vi "log analysis_gps.vi"() -> ()   [LabVIEW 2018] (continued)
41.292312622,-13.761383057,0.0,1.487377644,3.398363352,\"631T\",25,10,10,8,04,00,30,03*49b52b61\n\t", "INSPVAXA,USB3,0,44.5,FINESTEERING,2107,281284.250,02000000,471d,15824;INS_ALIGNMENT_COMPLETE,INS_RTKFIXED,37.37058446322,126.72127677415,9.0328,22.3000,0.3259,0.3273,-0.0037,-0.937814691,-0.658439283,39.092377906,0.4304,0.3133,0.6248,0.1182,0.0996,0.0951,0.2734,0.2534,5.0568,0f000001,0*6df0d0a0\n\t", "DUALANTENNAHEADINGA,USB3,0,45.0,FINESTEERING,2107,281285.200,02000000,d426,15824;SOL_COMPUTED,NARROW_INT,-1.000000000,40.100524902,-11.947021484,0.0,1.414593220,3.733982325,\"631T\",25,10,10,8,04,00,30,03*9b9ac519\n\t", "INSPVAXA,USB3,0,45.0,FINESTEERING,2107,281285.750,02000000,471d,15824;INS_ALIGNMENT_COMPLETE,INS_RTKFIXED,37.37058925318,126.72128198037,9.0239,22.3000,0.3334,0.2935,0.0143,-0.808488626,-0.666784324,37.099598741,0.4334,0.3188,0.6428,0.1170,0.0987,0.0941,0.2735,0.2534,5.0574,0f000001,0*332dca9d\n\t", "DUALANTENNAHEADINGA,USB3,0,47.0,FINESTEERING,2107,281286.700,02000000,d426,15824;SOL_COMPUTED,NARROW_INT,-1.000000000,38.718589783,-13.239685059,0.0,1.092944860,2.696835995,\"631T\",24,10,10,8,04,00,30,03*03484901\n\t", "DUALANTENNAHEADINGA,USB3,0,47.0,FINESTEERING,2107,281287.700,02000000,d426,15824;SOL_COMPUTED,NARROW_INT,-1.000000000,36.104297638,-13.498443604,0.0,0.922848761,2.195329189,\"631T\",26,10,10,8,04,00,30,03*04480a52\n\t", "INSPVAXA,USB3,0,47.5,FINESTEERING,2107,281288.250,02000000,471d,15824;INS_ALIGNMENT_COMPLETE,INS_RTKFIXED,37.37059781001,126.72128984433,9.0038,22.3000,0.3744,0.2594,-0.0022,-0.807848341,-0.697649833,32.607000206,0.4351,0.3197,0.6721,0.1156,0.0982,0.0924,0.2733,0.2531,5.0607,0f000001,0*7ad3d381\n\t", "DUALANTENNAHEADINGA,USB3,0,47.5,FINESTEERING,2107,281288.700,02000000,d426,15824;SOL_COMPUTED,NARROW_INT,-1.000000000,34.380798340,-12.289306641,0.0,0.881599903,2.027381897,\"631T\",24,10,10,8,04,00,30,03*fd23ace1\n\t", "INSPVAXA,USB3,0,43.0,FINESTEERING,2107,281289.250,02000000,471d,15824;INS_ALIGNMENT_COMPLETE,INS_RTKFIXED,37.37060144846,126.72129278207,8.9959,22.3000,0.3637,0.2540,-0.0055,-0.784801364,-1.198337190,31.676492197,0.4344,0.3185,0.6737,0.1148,0.0977,0.0905,0.2732,0.2529,5.0623,0f000001,0*0e64d244\n\t", "DUALANTENNAHEADINGA,USB3,0,47.0,FINESTEERING,2107,281290.200,02000000,d426,15824;SOL_COMPUTED,NARROW_INT,-1.000000000,34.493209839,-14.783813477,0.0,0.972535849,1.987741113,\"631T\",22,10,10,8,04,00,30,03*2d07aef6\n\t", "INSPVAXA,USB3,0,47.0,FINESTEERING,2107,281291.250,02000000,471d,15824;INS_ALIGNMENT_COMPLETE,INS_RTKFIXED,37.37060884718,126.72129871265,8.9767,22.3000,0.3938,0.2598,0.0143,-0.672164734,-1.279451684,31.580297519,0.4248,0.3046,0.6381,0.1143,0.0969,0.0864,0.2729,0.2527,5.0655,0f000001,0*eac27b45\n\t", "INSPVAXA,USB3,0,48.0,FINESTEERING,2107,281292.250,02000000,471d,15824;INS_ALIGNMENT_COMPLETE,INS_RTKFIXED,37.37061243778,126.72130169584,8.9693,22.3000,0.3929,0.2526,0.0002,-0.566566315,-1.022014825,31.866570439,0.4222,0.3014,0.6236,0.1151,0.0976,0.0859,0.2728,0.2526,5.0668,0f000001,0*f1faa83c\n\t", "INSPVAXA,USB3,0,46.5,FINESTEERING,2107,281293.250,02008000,471d,15824;INS_ALIGNMENT_COMPLETE,INS_RTKFIXED,37.37061609007,126.72130472150,8.9616,22.3000,0.3940,0.2710,0.0085,-0.635134028,-1.458627956,32.227180658,0.4201,0.2993,0.6101,0.1147,0.0971,0.0842,0.2727,0.2523,5.0683,0f000001,0*f561f230\n\t", "INSPVAXA,USB3,0,44.0,FINESTEERING,2107,281294.250,02008000,471d,15824;INS_ALIGNMENT_COMPLETE,INS_RTKFIXED,37.37061971209,126.72130780942,8.9541,22.3000,0.4211,0.2805,-0.0013,-0.831057528,-0.973116306,32.803325503,0.4188,0.2977,0.5988,0.1153,0.0975,0.0844,0.2725,0.2520,5.0696,0f000001,0*1928a823\n\t", "INSPVAXA,USB3,0,44.0,FINESTEERING,2107,281294.750,02008000,471d,15824;INS_ALIGNMENT_COMPLETE,INS_RTKFIXED,37.37062151019,126.72130936764,8.9520,22.3000,0.3975,0.2634,0.0090,-0.724790685,-1.060395947,33.026627760,0.4188,0.2977,0.5988,0.1153,0.0975,0.0844,0.2725,0.2520,5.0696,0f000001,0*daa7d020\n\t", "INSPVAXA,USB3,0,48.0,FINESTEERING,2107,281295.250,02008000,471d,15824;INS_ALIGNMENT_COMPLETE,INS_RTKFIXED,37.37062331676,126.72131094056,8.9508,22.3000,0.4136,0.2984,0.0031,-0.941558155,-1.233075222,33.345568477,0.4178,0.2964,0.5888,0.1164,0.0983,0.0857,0.2723,0.2516,5.0710,0f000001,0*4b91ac30\n\t", "INSPVAXA,USB3,0,48.0,FINESTEERING,2107,281295.750,02008000,471d,15824;INS_ALIGNMENT_COMPLETE,INS_RTKFIXED,37.37062507494,126.72131254716,8.9509,22.3000,0.4055,0.2849,-0.0018,-0.776132833,-1.125745955,33.718162525,0.4178,0.2964,0.5888,0.1164,0.0983,0.0857,0.2723,0.2516,5.0710,0f000001,0*fb568b3d\n\t", "INSPVAXA,USB3,0,46.0,FINESTEERING,2107,281296.750,02008000,471d,15824;INS_ALIGNMENT_COMPLETE,INS_RTKFIXED,37.37062859977,126.72131581022,8.9479,22.3000,0.4084,0.2870,-0.0048,-0.626858004,-1.220047276,34.496993035,0.4174,0.2953,0.5808,0.1166,0.0980,0.0866,0.2720,0.2512,5.0719,0f000001,0*b70d9a1a\n\t", "INSPVAXA,USB3,0,46.5,FINESTEERING,2107,281297.750,02000000,471d,15824;INS_ALIGNMENT_COMPLETE,INS_RTKFIXED,37.37063201269,126.72131910032,8.9415,22.3000,0.3858,0.2920,-0.0049,-0.857107455,-1.040274472,35.314316198,0.4170,0.2951,0.5749,0.1163,0.0975,0.0871,0.2718,0.2508,5.0734,0f000001,0*148bd1ed\n\t", "INSPVAXA,USB3,0,47.5,FINESTEERING,2107,281298.250,02000000,471d,15824;INS_ALIGNMENT_COMPLETE,INS_RTKFIXED,37.37063371305,126.72132080320,8.9374,22.3000,0.3749,0.3041,0.0076,-0.820490736,-1.287497218,35.568330559,0.4168,0.2950,0.5704,0.1159,0.0968,0.0877,0.2716,0.2505,5.0751,0f000001,0*0458b711\n\t", "INSPVAXA,USB3,0,48.0,FINESTEERING,2107,281299.250,02000000,471d,15824;INS_ALIGNMENT_COMPLETE,INS_RTKFIXED,37.37063695179,126.72132414290,8.9320,22.3000,0.3767,0.2972,0.0004,-0.739787726,-1.092581403,36.370475984,0.4162,0.2936,0.5661,0.1155,0.0962,0.0881,0.2714,0.2503,5.0767,0f000001,0*980b2911\n\t", "INSPVAXA,USB3,0,48.0,FINESTEERING,2107,281299.750,02000000,471d,15824;INS_ALIGNMENT_COMPLETE,INS_RTKFIXED,37.37063857725,126.72132585702,8.9270,22.3000,0.3719,0.3148,0.0043,-0.737895433,-1.223503382,36.673164573,0.4162,0.2936,0.5661,0.1155,0.0962,0.0881,0.2714,0.2503,5.0767,0f000001,0*b3e17f59\n\t", "INSPVAXA,USB3,0,49.0,FINESTEERING,2107,281300.750,02000000,471d,15824;INS_ALIGNMENT_COMPLETE,INS_RTKFIXED,37.37064174008,126.72132926537,8.9257,22.3000,0.3670,0.3118,0.0263,-0.579154984,-1.155742554,37.154805631,0.4158,0.2925,0.5630,0.1150,0.0956,0.0882,0.2713,0.2501,5.0783,0f000001,0*68bc3ddc\n\t", "INSPVAXA,USB3,0,45.0,FINESTEERING,2107,281301.250,02000000,471d,15824;INS_ALIGNMENT_COMPLETE,INS_RTKFIXED,37.37064333082,126.72133100341,8.9247,22.3000,0.3527,0.3031,-0.0127,-0.497881358,-1.036001571,37.376921117,0.4148,0.2915,0.5607,0.1142,0.0949,0.0876,0.2713,0.2501,5.0798,0f000001,0*cc5b3be5\n\t", "INSPVAXA,USB3,0,45.0,FINESTEERING,2107,281301.750,02000000,471d,15824;INS_ALIGNMENT_COMPLETE,INS_RTKFIXED,37.37064493780,126.72133275728,8.9253,22.3000,0.3854,0.3385,0.0182,-0.710763473,-1.064044201,37.431956874,0.4148,0.2915,0.5607,0.1142,0.0949,0.0876,0.2713,0.2501,5.0798,0f000001,0*85706bc5\n\t", "INSPVAXA,USB3,0,43.5,FINESTEERING,2107,281302.250,02000000,471d,15824;INS_ALIGNMENT_COMPLETE,INS_RTKFIXED,37.37064655535,126.72133453652,8.9249,22.3000,0.3513,0.3141,0.0174,-0.690110515,-1.069032412,37.638808056,0.4139,0.2898,0.5573,0.1136,0.0942,0.0868,0.2712,0.2501,5.0809,0f000001,0*cbae559e\n\t", "INSPVAXA,USB3,0,43.5,FINESTEERING,2107,281302.750,02000000,471d,15824;INS_ALIGNMENT_COMPLETE,INS_RTKFIXED,37.37064813520,126.72133627740,8.9245,22.3000,0.3692,0.3319,0.0061,-0.364312615,-0.951644319,37.470597230,0.4139,0.2898,0.5573,0.1136,0.0942,0.0868,0.2712,0.2501,5.0809,0f000001,0*08b0ee33\n\t", "INSPVAXA,USB3,0,47.5,FINESTEERING,2107,281303.750,02000000,471d,15824;INS_ALIGNMENT_COMPLETE,INS_RTKFIXED,37.37065132406,126.72133969488,8.9195,22.3000,0.3562,0.2992,-0.0320,-0.568216289,-0.963941072,36.278443582,0.4132,0.2892,0.5557,0.1134,0.0941,0.0862,0.2712,0.2500,5.0819,0f000001,0*4328ab23\n\t", "INSPVAXA,USB3,0,48.0,FINESTEERING,2107,281304.250,02000000,471d,15824;INS_ALIGNMENT_COMPLETE,INS_RTKFIXED,37.37065295180,126.72134135022,8.9157,22.3000,0.3763,0.3181,0.0214,-0.552058528,-1.148423815,35.386724637,0.4128,0.2880,0.5530,0.1133,0.0938,0.0856,0.2712,0.2500,5.0827,0f000001,0*325fffc2\n\t", "INSPVAXA,USB3,0,49.0,FINESTEERING,2107,281305.250,02000000,471d,15824;INS_ALIGNMENT_COMPLETE,INS_RTKFIXED,37.37065630183,126.72134454819,8.9059,22.3000,0.3906,0.3004,-0.0040,-0.611614094,-1.196662940,33.418986563,0.4115,0.2871,0.5504,0.1130,0.0936,0.0850,0.2711,0.2499,5.0838,0f000001,0*b360f959\n\t", "INSPVAXA,USB3,0,49.0,FINESTEERING,2107,281305.750,02000000,471d,15824;INS_ALIGNMENT_COMPLETE,INS_RTKFIXED,37.37065799694,126.72134610571,8.8988,22.3000,0.3773,0.2695,-0.0206,-0.928046219,-1.204880173,32.568917914,0.4115,0.2871,0.5504,0.1130,0.0936,0.0850,0.2711,0.2499,5.0838,0f000001,0*cfbde854\n\t", "INSPVAXA,USB3,0,43.0,FINESTEERING,2107,281306.750,02000000,471d,15824;INS_ALIGNMENT_COMPLETE,INS_RTKFIXED,37.37066149033,126.72134911698,8.8812,22.3000,0.3665,0.2586,0.0068,-0.726996907,-1.292564027,31.229501347,0.4104,0.2857,0.5476,0.1128,0.0935,0.0845,0.2710,0.2498,5.0853,0f000001,0*271f73c6\n\t", "INSPVAXA,USB3,0,47.5,FINESTEERING,2107,281307.250,02000000,471d,15824;INS_ALIGNMENT_COMPLETE,INS_RTKFIXED,37.37066326651,126.72135056496,8.8706,22.3000,0.3793,0.2759,-0.0087,-0.800097875,-1.188494571,30.825604162,0.4094,0.2846,0.5448,0.1127,0.0934,0.0841,0.2709,0.2497,5.0869,0f000001,0*7a768f4f\n\t", "INSPVAXA,USB3,0,47.5,FINESTEERING,2107,281307.750,02000000,471d,15824;INS_ALIGNMENT_COMPLETE,INS_RTKFIXED,37.37066506990,126.72135204695,8.8605,22.3000,0.3836,0.2569,-0.0181,-0.611818714,-1.092696034,30.573284565,0.4094,0.2846,0.5448,0.1127,0.0934,0.0841,0.2709,0.2497,5.0869,0f000001,0*79d635a4\n\t", "INSPVAXA,USB3,0,46.0,FINESTEERING,2107,281308.250,02000000,471d,15824;INS_ALIGNMENT_COMPLETE,INS_RTKFIXED,37.37066685186,126.72135349986,8.8501,22.3000,0.3922,0.2593,-0.0136,-0.551675825,-0.866778153,30.503806411,0.4391,0.2876,0.5552,0.1178,0.0942,0.0847,0.2709,0.2501,5.0885,0f000001,0*c2dc3b9a\n\t", "INSPVAXA,USB3,0,46.0,FINESTEERING,2107,281308.750,02000000,471d,15824;INS_ALIGNMENT_COMPLETE,INS_RTKFIXED,37.37066865801,126.72135498437,8.8428,22.3000,0.3889,0.2874,-0.0164,-0.422088252,-1.035305211,30.456393421,0.4391,0.2876,0.5552,0.1178,0.0942,0.0847,0.2709,0.2501,5.0885,0f000001,0*b848ab12\n\t", "INSPVAXA,USB3,0,48.0,FINESTEERING,2107,281309.750,02000000,471d,15824;INS_ALIGNMENT_COMPLETE,INS_RTKFIXED,37.37067230614,126.72135792146,8.8292,22.3000,0.4110,0.2664,-0.0105,-0.611662697,-1.081629993,30.781825564,0.4668,0.2909,0.5674,0.1216,0.0948,0.0853,0.2709,0.2504,5.0902,0f000001,0*6b834f48\n\t", "INSPVAXA,USB3,0,46.5,FINESTEERING,2107,281310.250,02000000,471d,15824;INS_ALIGNMENT_COMPLETE,INS_RTKFIXED,37.37067411015,126.72135939117,8.8212,22.3000,0.3810,0.2710,-0.0053,-0.603115000,-1.192069099,31.016227995,0.4406,0.2869,0.5568,0.1163,0.0939,0.0842,0.2707,0.2496,5.0919,0f000001,0*94346154\n\t", "INSPVAXA,USB3,0,46.5,FINESTEERING,2107,281310.750,02000000,471d,15824;INS_ALIGNMENT_COMPLETE,INS_RTKFIXED,37.37067588400,126.72136084983,8.8127,22.3000,0.4076,0.2839,-0.0115,-0.606845317,-1.152685391,31.227730506,0.4406,0.2869,0.5568,0.1163,0.0939,0.0842,0.2707,0.2496,5.0919,0f000001,0*103e46f3\n\t", "INSPVAXA,USB3,0,46.5,FINESTEERING,2107,281311.250,02000000,471d,15824;INS_ALIGNMENT_COMPLETE,INS_RTKFIXED,37.37067773364,126.72136238370,8.8047,22.3000,0.4077,0.2865,0.0068,-0.584908191,-1.091980758,31.544161154,0.4259,0.2849,0.5501,0.1143,0.0937,0.0835,0.2705,0.2492,5.0936,0f000001,0*c1eb006b\n\t", "INSPVAXA,USB3,0,46.5,FINESTEERING,2107,281311.750,02000000,471d,15824;INS_ALIGNMENT_COMPLETE,INS_RTKFIXED,37.37067959251,126.72136394573,8.7964,22.3000,0.4141,0.2904,-0.0295,-0.451303180,-1.068459528,31.726821051,0.4259,0.2849,0.5501,0.1143,0.0937,0.0835,0.2705,0.2492,5.0936,0f000001,0*f5652221\n\t", "INSPVAXA,USB3,0,48.5,FINESTEERING,2107,281312.250,02000000,471d,15824;INS_ALIGNMENT_COMPLETE,INS_RTKFIXED,37.37068138188,126.72136546046,8.7891,22.3000,0.3907,0.2897,-0.0164,-0.536773748,-1.064691543,31.954893776,0.4173,0.2841,0.5455,0.1136,0.0938,0.0834,0.2704,0.2490,5.0951,0f000001,0*3086f5e7\n\t", "INSPVAXA,USB3,0,48.5,FINESTEERING,2107,281312.750,02000000,471d,15824;INS_ALIGNMENT_COMPLETE,INS_RTKFIXED,37.37068318728,126.72136703307,8.7806,22.3000,0.4101,0.2924,-0.0105,-0.304454074,-0.851881109,32.302829580,0.4173,0.2841,0.5455,0.1136,0.0938,0.0834,0.2704,0.2490,5.0951,0f000001,0*5034c2f1\n\t", "INSPVAXA,USB3,0,45.5,FINESTEERING,2107,281314.250,02000000,471d,15824;INS_ALIGNMENT_COMPLETE,INS_RTKFIXED,37.37068860278,126.72137185474,8.7599,22.3000,0.3783,0.2883,-0.0099,-0.473451897,-1.199118445,33.419872159,0.4114,0.2852,0.5433,0.1126,0.0924,0.0813,0.2701,0.2485,5.0982,0f000001,0*254465a8\n\t", "INSPVAXA,USB3,0,45.5,FINESTEERING,2107,281314.750,02000000,471d,15824;INS_ALIGNMENT_COMPLETE,INS_RTKFIXED,37.37069038063,126.72137348955,8.7529,22.3000,0.4019,0.3010,-0.0013,-0.576554942,-1.350073245,33.962253064,0.4114,0.2852,0.5433,0.1126,0.0924,0.0813,0.2701,0.2485,5.0982,0f000001,0*70de1d9e\n\t", "INSPVAXA,USB3,0,50.0,FINESTEERING,2107,281316.250,02000000,471d,15824;INS_ALIGNMENT_COMPLETE,INS_RTKFIXED,37.37069553748,126.72137835296,8.7291,22.3000,0.3690,0.3016,-0.0165,-0.475362397,-1.709507066,35.267633649,0.4099,0.2844,0.5412,0.1123,0.0915,0.0796,0.2698,0.2480,5.0999,0f000001,0*7a9fb179\n\t", "INSPVAXA,USB3,0,50.5,FINESTEERING,2107,281317.250,02000000,471d,15824;INS_ALIGNMENT_COMPLETE,INS_RTKFIXED,37.37069888473,126.72138166049,8.7140,22.3000,0.4002,0.3322,-0.0336,-0.163313359,-1.347458535,36.032748786,0.4094,0.2836,0.5396,0.1129,0.0921,0.0802,0.2696,0.2478,5.0996,0f000001,0*7e476d51\n\t", "INSPVAXA,USB3,0,50.0,FINESTEERING,2107,281318.250,02000000,471d,15824;INS_ALIGNMENT_COMPLETE,INS_RTKFIXED,37.37070219067,126.72138499710,8.7014,22.3000,0.3959,0.3213,-0.0090,-0.394966992,-1.322496913,36.727773169,0.4088,0.2828,0.5369,0.1123,0.0917,0.0794,0.2695,0.2477,5.0989,0f000001,0*0ac65207\n\t", "INSPVAXA,USB3,0,48.5,FINESTEERING,2107,281319.750,02000000,471d,15824;INS_ALIGNMENT_COMPLETE,INS_RTKFIXED,37.37070705981,126.72139005862,8.6887,22.3000,0.3656,0.3184,-0.0246,-0.462020881,-1.503034844,37.411185291,0.4083,0.2820,0.5343,0.1120,0.0915,0.0787,0.2694,0.2475,5.0983,0f000001,0*abb76b38\n\t", "INSPVAXA,USB3,0,48.5,FINESTEERING,2107,281320.750,02000000,471d,15824;INS_ALIGNMENT_COMPLETE,INS_RTKFIXED,37.37071031528,126.72139346401,8.6801,22.3000,0.3719,0.3343,-0.0256,-0.836621928,-1.161971448,37.866051675,0.4083,0.2824,0.5333,0.1117,0.0916,0.0783,0.2693,0.2474,5.0979,0f000001,0*4c0e47a3\n\t", "INSPVAXA,USB3,0,47.0,FINESTEERING,2107,281322.250,02000000,471d,15824;INS_ALIGNMENT_COMPLETE,INS_RTKFIXED,37.37071517986,126.72139865405,8.6652,22.3000,0.3760,0.3375,-0.0171,-0.655763747,-1.033016654,37.379702834,0.4086,0.2835,0.5329,0.1123,0.0925,0.0785,0.2691,0.2470,5.0988,0f000001,0*f362831b\n\t", "INSPVAXA,USB3,0,48.5,FINESTEERING,2107,281323.750,02000000,471d,15824;INS_ALIGNMENT_COMPLETE,INS_RTKFIXED,37.37072004459,126.72140359087,8.6528,22.3000,0.3627,0.2855,-0.0006,-0.403703824,-0.919601594,35.267300347,0.4085,0.2834,0.5316,0.1119,0.0920,0.0781,0.2688,0.2467,5.1000,0f000001,0*ec9c6181\n\t", "INSPVAXA,USB3,0,48.0,FINESTEERING,2107,281350.300,02000000,471d,15824;INS_ALIGNMENT_COMPLETE,INS_RTKFIXED,37.37080986573,126.72148875740,8.5075,22.3000,0.3628,0.2976,-0.0057,-1.206867274,-0.983762536,33.908435264,0.4194,0.3028,0.5790,0.1129,0.0949,0.0832,0.2672,0.2431,5.1219,0f000001,0*073b2b30\n\t", "INSPVAXA,USB3,0,48.0,FINESTEERING,2107,281351.800,02000000,471d,15824;INS_ALIGNMENT_COMPLETE,INS_RTKFIXED,37.37081508694,126.72149360654,8.4972,22.3000,0.3531,0.2937,-0.0017,-1.250896951,-0.823004101,34.091002532,0.4207,0.3049,0.5833,0.1126,0.0947,0.0826,0.2672,0.2430,5.1224,0f000001,0*3c5ad9c3\n\t", "INSPVAXA,USB3,0,49.0,FINESTEERING,2107,281355.800,02000000,471d,15824;INS_ALIGNMENT_COMPLETE,INS_RTKFIXED,37.37082893700,126.72150664306,8.4666,22.3000,0.3730,0.3109,-0.0009,-1.161970784,-1.138060141,34.996264200,0.4190,0.3015,0.5793,0.1125,0.0944,0.0820,0.2670,0.2425,5.1250,0f000001,0*10c36a68\n\t", "INSPVAXA,USB3,0,48.0,FINESTEERING,2107,281356.300,02000000,471d,15824;INS_ALIGNMENT_COMPLETE,INS_RTKFIXED,37.37083063572,126.72150829045,8.4620,22.3000,0.3521,0.3106,-0.0162,-1.118678244,-0.900069608,35.100092302,0.4187,0.3015,0.5781,0.1134,0.0955,0.0834,0.2669,0.2424,5.1261,0f000001,0*ecce3653\n\t", "INSPVAXA,USB3,0,48.0,FINESTEERING,2107,281356.800,02000000,471d,15824;INS_ALIGNMENT_COMPLETE,INS_RTKFIXED,37.37083231067,126.72150995992,8.4554,22.3000,0.3495,0.3060,0.0042,-0.932722694,-0.812097133,35.195809963,0.4187,0.3015,0.5781,0.1134,0.0955,0.0834,0.2669,0.2424,5.1261,0f000001,0*f7e2c3ce\n\t", "INSPVAXA,USB3,0,47.5,FINESTEERING,2107,281358.300,02000000,471d,15824;INS_ALIGNMENT_COMPLETE,INS_RTKFIXED,37.37083738053,126.72151493365,8.4383,22.3000,0.3581,0.3251,0.0034,-0.998984174,-0.973141435,35.285574115,0.4158,0.2963,0.5677,0.1128,0.0943,0.0826,0.2668,0.2421,5.1287,0f000001,0*5ae881cd\n\t", "INSPVAXA,USB3,0,47.5,FINESTEERING,2107,281358.800,02000000,471d,15824;INS_ALIGNMENT_COMPLETE,INS_RTKFIXED,37.37083909479,126.72151662067,8.4311,22.3000,0.3558,0.3072,-0.0005,-0.868229023,-1.222380492,35.266513132,0.4158,0.2963,0.5677,0.1128,0.0943,0.0826,0.2668,0.2421,5.1287,0f000001,0*f5ce0274\n\t", "DUALANTENNAHEADINGA,USB3,0,49.0,FINESTEERING,2107,281360.300,02000000,d426,15824;SOL_COMPUTED,NARROW_FLOAT,-1.000000000,43.377029419,-28.936859131,0.0,317.200378418,180.000000000,\"631T\",19,9,9,8,04,00,20,03*d052c393\n\t", "DUALANTENNAHEADINGA,USB3,0,49.0,FINESTEERING,2107,281360.800,02000000,d426,15824;SOL_COMPUTED,NARROW_FLOAT,-1.000000000,41.997791290,-30.735473633,0.0,321.670349121,180.000000000,\"631T\",18,9,9,8,04,00,20,03*cef783d0\n\t", "DUALANTENNAHEADINGA,USB3,0,46.5,FINESTEERING,2107,281361.300,02000000,d426,15824;SOL_COMPUTED,NARROW_FLOAT,-1.000000000,39.328605652,-30.210357666,0.0,354.292755127,180.000000000,\"631T\",19,9,9,8,04,00,20,03*65c8eaaf\n\t", "INSPVAXA,USB3,0,46.5,FINESTEERING,2107,281361.800,02000000,471d,15824;INS_ALIGNMENT_COMPLETE,INS_RTKFIXED,37.37084928466,126.72152648987,8.4001,22.3000,0.3666,0.2894,0.0007,-0.918254878,-1.223429977,34.701580667,0.4179,0.3011,0.5737,0.1121,0.0941,0.0814,0.2668,0.2419,5.1323,0f000001,0*40ddb97a\n\t", "DUALANTENNAHEADINGA,USB3,0,48.0,FINESTEERING,2107,281362.300,02000000,d426,15824;SOL_COMPUTED,NARROW_FLOAT,-1.000000000,51.965854645,-24.394927979,0.0,236.640274048,180.000000000,\"631T\",19,9,9,8,04,00,20,03*62047533\n\t", "DUALANTENNAHEADINGA,USB3,0,48.0,FINESTEERING,2107,281362.800,02000000,d426,15824;SOL_COMPUTED,NARROW_FLOAT,-1.000000000,51.700309753,-22.485168457,0.0,233.081008911,180.000000000,\"631T\",19,9,9,8,04,00,20,03*ce0df6af\n\t", "DUALANTENNAHEADINGA,USB3,0,46.0,FINESTEERING,2107,281363.300,02000000,d426,15824;SOL_COMPUTED,NARROW_FLOAT,-1.000000000,37.930927277,-27.303833008,0.0,334.334472656,180.000000000,\"631T\",20,9,9,7,04,00,20,03*296cd207\n\t", "DUALANTENNAHEADINGA,USB3,0,46.0,FINESTEERING,2107,281363.800,02000000,d426,15824;SOL_COMPUTED,NARROW_FLOAT,-1.000000000,38.201625824,-27.727355957,0.0,332.017791748,180.000000000,\"631T\",23,9,9,8,04,00,20,03*f0493f23\n\t", "DUALANTENNAHEADINGA,USB3,0,44.0,FINESTEERING,2107,281364.300,02000000,d426,15824;SOL_COMPUTED,NARROW_FLOAT,-1.000000000,49.235725403,-25.915039063,0.0,256.086944580,180.000000000,\"631T\",24,9,9,8,04,00,20,03*6ae9d837\n\t", "INSPVAXA,USB3,0,44.0,FINESTEERING,2107,281364.800,02000000,471d,15824;INS_ALIGNMENT_COMPLETE,INS_RTKFIXED,37.37085965164,126.72153621397,8.3672,22.3000,0.3702,0.3004,-0.0120,-0.629392429,-1.475289805,34.330847261,0.4175,0.2991,0.5747,0.1118,0.0936,0.0803,0.2665,0.2416,5.1319,0f000001,0*907d57c4\n\t", "DUALANTENNAHEADINGA,USB3,0,48.0,FINESTEERING,2107,281365.300,02000000,d426,15824;SOL_COMPUTED,NARROW_FLOAT,-1.000000000,46.742221832,-24.611022949,0.0,308.216918945,180.000000000,\"631T\",18,9,9,8,04,00,20,03*16f83fc7\n\t", "DUALANTENNAHEADINGA,USB3,0,48.0,FINESTEERING,2107,281365.800,02000000,d426,15824;SOL_COMPUTED,NARROW_FLOAT,-1.000000000,45.876544952,-25.206176758,0.0,301.727966309,180.000000000,\"631T\",19,9,9,8,04,00,20,03*878e3cfa\n\t", "INSPVAXA,USB3,0,50.0,FINESTEERING,2107,281366.300,02000000,471d,15824;INS_ALIGNMENT_COMPLETE,INS_RTKFIXED,37.37086481879,126.72154103574,8.3492,22.3000,0.3841,0.2933,-0.0130,-0.540868347,-1.307063717,34.323850336,0.4168,0.2979,0.5715,0.1114,0.0932,0.0794,0.2664,0.2414,5.1301,0f000001,0*c00b2394\n\t", "INSPVAXA,USB3,0,50.0,FINESTEERING,2107,281366.800,02000000,471d,15824;INS_ALIGNMENT_COMPLETE,INS_RTKFIXED,37.37086653652,126.72154262606,8.3447,22.3000,0.3779,0.3041,-0.0177,-0.586317091,-1.274041965,34.268661727,0.4168,0.2979,0.5715,0.1114,0.0932,0.0794,0.2664,0.2414,5.1301,0f000001,0*197e2cdd\n\t", "DUALANTENNAHEADINGA,USB3,0,48.0,FINESTEERING,2107,281367.300,02000000,d426,15824;SOL_COMPUTED,NARROW_FLOAT,-1.000000000,57.061241150,-31.246337891,0.0,140.264724731,180.000000000,\"631T\",19,11,11,8,04,00,30,03*83af5acf\n\t", "DUALANTENNAHEADINGA,USB3,0,48.0,FINESTEERING,2107,281367.800,02000000,d426,15824;SOL_COMPUTED,NARROW_FLOAT,-1.000000000,57.968719482,-32.427215576,0.0,139.111709595,180.000000000,\"631T\",22,11,11,8,04,00,30,03*64b77029\n\t", "INSPVAXA,USB3,0,45.0,FINESTEERING,2107,281368.300,02000000,471d,15824;INS_ALIGNMENT_COMPLETE,INS_RTKFIXED,37.37087168794,126.72154735160,8.3372,22.3000,0.3761,0.3168,-0.0092,-0.837699273,-0.815511230,34.270342618,0.4149,0.2944,0.5637,0.1114,0.0930,0.0792,0.2662,0.2411,5.1296,0f000001,0*cf514333\n\t", "INSPVAXA,USB3,0,45.0,FINESTEERING,2107,281368.800,02000000,471d,15824;INS_ALIGNMENT_COMPLETE,INS_RTKFIXED,37.37087344572,126.72154897754,8.3331,22.3000,0.3716,0.2920,0.0040,-0.667583562,-0.920128671,34.279798590,0.4149,0.2944,0.5637,0.1114,0.0930,0.0792,0.2662,0.2411,5.1296,0f000001,0*f456fa2a\n\t", "DUALANTENNAHEADINGA,USB3,0,47.0,FINESTEERING,2107,281369.300,02000000,d426,15824;SOL_COMPUTED,NARROW_FLOAT,-1.000000000,48.869911194,-23.291656494,0.0,246.362884521,180.000000000,\"631T\",19,9,9,8,04,00,20,03*fdb2b4cf\n\t", "INSPVAXA,USB3,0,47.0,FINESTEERING,2107,281369.800,02000000,471d,15824;INS_ALIGNMENT_COMPLETE,INS_RTKFIXED,37.37087693639,126.72155218192,8.3258,22.3000,0.3824,0.3082,-0.0032,-0.585559020,-1.104223780,34.420056753,0.4144,0.2935,0.5605,0.1112,0.0927,0.0788,0.2662,0.2410,5.1304,0f000001,0*fed5d425\n\t", "DUALANTENNAHEADINGA,USB3,0,48.5,FINESTEERING,2107,281370.300,02000000,d426,15824;SOL_COMPUTED,NARROW_FLOAT,-1.000000000,56.995876312,-45.029174805,0.0,226.826354980,180.000000000,\"631T\",18,8,8,8,04,00,20,03*06abc766\n\t", "DUALANTENNAHEADINGA,USB3,0,48.5,FINESTEERING,2107,281370.800,02000000,d426,15824;SOL_COMPUTED,NARROW_FLOAT,-1.000000000,56.755435944,-45.314361572,0.0,225.346038818,180.000000000,\"631T\",19,8,8,8,04,00,20,03*c8312a5e\n\t", "DUALANTENNAHEADINGA,USB3,0,47.5,FINESTEERING,2107,281371.800,02000000,d426,15824;SOL_COMPUTED,NARROW_FLOAT,-1.000000000,65.830406189,-48.192810059,0.0,160.190460205,180.000000000,\"631T\",20,8,8,8,04,00,20,03*a1e2e423\n\t", "DUALANTENNAHEADINGA,USB3,0,51.0,FINESTEERING,2107,281372.300,02000000,d426,15824;SOL_COMPUTED,NARROW_FLOAT,-1.000000000,46.303096771,-16.665802002,0.0,249.117385864,180.000000000,\"631T\",21,9,9,8,04,00,20,03*9ebf37bc\n\t", "DUALANTENNAHEADINGA,USB3,0,51.0,FINESTEERING,2107,281372.800,02000000,d426,15824;SOL_COMPUTED,NARROW_FLOAT,-1.000000000,47.137203217,-16.407073975,0.0,245.953109741,180.000000000,\"631T\",21,9,9,8,04,00,20,03*e468614e\n\t", "DUALANTENNAHEADINGA,USB3,0,48.0,FINESTEERING,2107,281373.300,02000000,d426,15824;SOL_COMPUTED,NARROW_FLOAT,-1.000000000,40.694911957,-17.624786377,0.0,282.511657715,180.000000000,\"631T\",21,9,9,8,04,00,20,03*fc4a9f69\n\t", "DUALANTENNAHEADINGA,USB3,0,48.0,FINESTEERING,2107,281373.800,02000000,d426,15824;SOL_COMPUTED,NARROW_FLOAT,-1.000000000,39.396804810,-18.797271729,0.0,283.153411865,180.000000000,\"631T\",22,9,9,8,04,00,20,03*8a178ec6\n\t", "DUALANTENNAHEADINGA,USB3,0,45.0,FINESTEERING,2107,281374.800,02000000,d426,15824;SOL_COMPUTED,NARROW_FLOAT,-1.000000000,39.349189758,-20.650939941,0.0,277.168212891,180.000000000,\"631T\",22,9,9,8,04,00,20,03*f8ab3252\n\t", "DUALANTENNAHEADINGA,USB3,0,44.5,FINESTEERING,2107,281375.300,02000000,d426,15824;SOL_COMPUTED,NARROW_FLOAT,-1.000000000,34.529243469,-20.115325928,0.0,317.339965820,180.000000000,\"631T\",22,9,9,8,04,00,20,03*a594d36f\n\t", "DUALANTENNAHEADINGA,USB3,0,44.5,FINESTEERING,2107,281375.800,02000000,d426,15824;SOL_COMPUTED,NARROW_FLOAT,-1.000000000,34.753417969,-19.800323486,0.0,315.846893311,180.000000000,\"631T\",22,9,9,8,04,00,20,03*6b0303b2\n\t", "DUALANTENNAHEADINGA,USB3,0,46.0,FINESTEERING,2107,281376.300,02000000,d426,15824;SOL_COMPUTED,NARROW_FLOAT,-1.000000000,41.617706299,-20.286529541,0.0,249.996673584,180.000000000,\"631T\",22,9,9,8,04,00,20,03*8e0e78c9\n\t", "DUALANTENNAHEADINGA,USB3,0,45.0,FINESTEERING,2107,281377.300,02000000,d426,15824;SOL_COMPUTED,NARROW_FLOAT,-1.000000000,38.012714386,-20.573577881,0.0,307.964691162,180.000000000,\"631T\",20,9,9,8,04,00,20,03*3937b18a\n\t", "DUALANTENNAHEADINGA,USB3,0,45.0,FINESTEERING,2107,281377.800,02000000,d426,15824;SOL_COMPUTED,NARROW_FLOAT,-1.000000000,38.498992920,-20.027069092,0.0,303.899200439,180.000000000,\"631T\",20,9,9,8,04,00,20,03*e32a34d5\n\t", "DUALANTENNAHEADINGA,USB3,0,49.5,FINESTEERING,2107,281378.300,02000000,d426,15824;SOL_COMPUTED,NARROW_FLOAT,-1.000000000,27.239126205,-17.903564453,0.0,360.000000000,180.000000000,\"631T\",20,9,9,8,04,00,20,03*3fff5ac6\n\t", "DUALANTENNAHEADINGA,USB3,0,48.5,FINESTEERING,2107,281379.300,02000000,d426,15824;SOL_COMPUTED,NARROW_FLOAT,-1.000000000,30.153203964,-39.951202393,0.0,341.163116455,180.000000000,\"631T\",22,8,8,8,04,00,20,03*fe3aefcd\n\t", "DUALANTENNAHEADINGA,USB3,0,47.5,FINESTEERING,2107,281380.300,02000000,d426,15824;SOL_COMPUTED,NARROW_FLOAT,-1.000000000,31.592365265,-19.809661865,0.0,316.837921143,180.000000000,\"631T\",19,9,9,8,04,00,20,03*09fa2adc\n\t", "DUALANTENNAHEADINGA,USB3,0,46.0,FINESTEERING,2107,281381.300,02000000,d426,15824;SOL_COMPUTED,NARROW_FLOAT,-1.000000000,31.278856277,-21.390625000,0.0,327.912139893,180.000000000,\"631T\",19,9,9,8,04,00,20,03*4fc11f4c\n\t", "INSPVAXA,USB3,0,46.0,FINESTEERING,2107,281381.850,02000000,471d,15824;INS_ALIGNMENT_COMPLETE,INS_RTKFIXED,37.37091780548,126.72159081675,8.2350,22.3000,0.3759,0.2927,0.0016,-0.963689803,-1.123540768,33.630773348,0.4181,0.3018,0.5653,0.1129,0.0953,0.0850,0.2661,0.2404,5.1482,0f000001,0*05f2b425\n\t", "DUALANTENNAHEADINGA,USB3,0,49.5,FINESTEERING,2107,281382.800,02000000,d426,15824;SOL_COMPUTED,NARROW_FLOAT,-1.000000000,34.756454468,-17.411163330,0.0,292.158599854,180.000000000,\"631T\",19,9,9,8,04,00,20,03*833ed280\n\t", "DUALANTENNAHEADINGA,USB3,0,48.0,FINESTEERING,2107,281383.300,02000000,d426,15824;SOL_COMPUTED,NARROW_FLOAT,-1.000000000,29.882240295,-12.166564941,0.0,299.295318604,180.000000000,\"631T\",20,9,9,8,04,00,20,03*2118f19e\n\t", "INSPVAXA,USB3,0,48.0,FINESTEERING,2107,281383.850,02000000,471d,15824;INS_ALIGNMENT_COMPLETE,INS_RTKFIXED,37.37092469082,126.72159717751,8.2117,22.3000,0.3710,0.2982,-0.0132,-1.063340683,-1.217564676,33.617373330,0.4191,0.3013,0.5725,0.1134,0.0950,0.0851,0.2661,0.2404,5.1497,0f000001,0*b9a6888a\n\t", "INSPVAXA,USB3,0,49.0,FINESTEERING,2107,281385.350,02000000,471d,15824;INS_ALIGNMENT_COMPLETE,INS_RTKFIXED,37.37092984687,126.72160192884,8.2009,22.3000,0.3659,0.2906,-0.0108,-0.966416737,-0.773960288,33.451430049,0.4185,0.2991,0.5729,0.1134,0.0948,0.0848,0.2660,0.2403,5.1498,0f000001,0*c2089fa9\n\t", "INSPVAXA,USB3,0,49.0,FINESTEERING,2107,281385.850,02000000,471d,15824;INS_ALIGNMENT_COMPLETE,INS_RTKFIXED,37.37093156972,126.72160349245,8.1991,22.3000,0.3552,0.2819,0.0017,-0.982402524,-0.987093830,33.457221519,0.4185,0.2991,0.5729,0.1134,0.0948,0.0848,0.2660,0.2403,5.1498,0f000001,0*8db597c9\n\t", "INSPVAXA,USB3,0,46.0,FINESTEERING,2107,281386.850,02000000,471d,15824;INS_ALIGNMENT_COMPLETE,INS_RTKFIXED,37.37093500656,126.72160657159,8.1978,22.3000,0.3860,0.2986,-0.0065,-0.930872832,-0.693352418,33.361120344,0.4182,0.2979,0.5715,0.1134,0.0948,0.0846,0.2660,0.2403,5.1494,0f000001,0*a8ec127a\n\t", "INSPVAXA,USB3,0,48.5,FINESTEERING,2107,281387.850,02000000,471d,15824;INS_ALIGNMENT_COMPLETE,INS_RTKFIXED,37.37093847805,126.72160977606,8.1934,22.3000,0.3545,0.2733,-0.0290,-0.871913936,-1.019858036,33.407520693,0.4181,0.2974,0.5707,0.1132,0.0948,0.0844,0.2660,0.2403,5.1492,0f000001,0*8b26d1b5\n\t", "INSPVAXA,USB3,0,47.0,FINESTEERING,2107,281388.850,02000000,471d,15824;INS_ALIGNMENT_COMPLETE,INS_RTKFIXED,37.37094185798,126.72161284652,8.1862,22.3000,0.3458,0.2807,0.0000,-0.647146834,-0.755815505,33.229882391,0.4177,0.2968,0.5693,0.1134,0.0951,0.0842,0.2659,0.2403,5.1493,0f000001,0*e04b9d7e\n\t", "INSPVAXA,USB3,0,51.0,FINESTEERING,2107,281389.850,02000000,471d,15824;INS_ALIGNMENT_COMPLETE,INS_RTKFIXED,37.37094531152,126.72161597043,8.1814,22.3000,0.3770,0.3007,-0.0075,-0.964998734,-0.610692019,33.331132112,0.4178,0.2983,0.5697,0.1133,0.0955,0.0841,0.2659,0.2402,5.1491,0f000001,0*f3e7f4f6\n\t", "INSPVAXA,USB3,0,50.5,FINESTEERING,2107,281390.350,02000000,471d,15824;INS_ALIGNMENT_COMPLETE,INS_RTKFIXED,37.37094699615,126.72161749721,8.1810,22.3000,0.3585,0.2781,-0.0176,-0.963426361,-0.735868518,33.269975778,0.4179,0.2987,0.5691,0.1132,0.0952,0.0837,0.2658,0.2402,5.1481,0f000001,0*d9e47fdc\n\t", "INSPVAXA,USB3,0,50.5,FINESTEERING,2107,281390.850,02000000,471d,15824;INS_ALIGNMENT_COMPLETE,INS_RTKFIXED,37.37094874032,126.72161908849,8.1805,22.3000,0.3294,0.2293,-0.0009,-0.908401670,-0.595727338,33.364278854,0.4179,0.2987,0.5691,0.1132,0.0952,0.0837,0.2658,0.2402,5.1481,0f000001,0*5999a9d2\n\t", "INSPVAXA,USB3,0,48.0,FINESTEERING,2107,281391.350,02000000,471d,15824;INS_ALIGNMENT_COMPLETE,INS_RTKFIXED,37.37095049924,126.72162069173,8.1796,22.3000,0.4034,0.3085,-0.0112,-0.795383493,-0.971346032,33.378242699,0.4182,0.2986,0.5686,0.1132,0.0949,0.0836,0.2658,0.2402,5.1464,0f000001,0*1e48eff8\n\t", "INSPVAXA,USB3,0,48.0,FINESTEERING,2107,281391.850,02000000,471d,15824;INS_ALIGNMENT_COMPLETE,INS_RTKFIXED,37.37095218768,126.72162223158,8.1782,22.3000,0.3736,0.3039,0.0085,-0.869440972,-1.042554722,33.323263236,0.4182,0.2986,0.5686,0.1132,0.0949,0.0836,0.2658,0.2402,5.1464,0f000001,0*be662b3c\n\t", "INSPVAXA,USB3,0,46.5,FINESTEERING,2107,281392.850,02000000,471d,15824;INS_ALIGNMENT_COMPLETE,INS_RTKFIXED,37.37095563956,126.72162543709,8.1738,22.3000,0.3750,0.2874,-0.0042,-0.381103782,-1.196591916,33.536451772,0.4182,0.2976,0.5666,0.1131,0.0944,0.0833,0.2657,0.2401,5.1446,0f000001,0*fd2c5164\n\t", "INSPVAXA,USB3,0,47.0,FINESTEERING,2107,281393.350,02000000,471d,15824;INS_ALIGNMENT_COMPLETE,INS_RTKFIXED,37.37095732903,126.72162695963,8.1710,22.3000,0.3684,0.2951,-0.0131,-0.615904330,-1.127921907,33.544859726,0.4171,0.2952,0.5633,0.1132,0.0946,0.0833,0.2656,0.2401,5.1445,0f000001,0*dbe231da\n\t", "INSPVAXA,USB3,0,47.0,FINESTEERING,2107,281393.850,02000000,471d,15824;INS_ALIGNMENT_COMPLETE,INS_RTKFIXED,37.37095908537,126.72162857603,8.1657,22.3000,0.3533,0.2801,-0.0216,-0.431209048,-1.265989093,33.662345403,0.4171,0.2952,0.5633,0.1132,0.0946,0.0833,0.2656,0.2401,5.1445,0f000001,0*22a3a0dc\n\t", "INSPVAXA,USB3,0,49.5,FINESTEERING,2107,281394.350,02000000,471d,15824;INS_ALIGNMENT_COMPLETE,INS_RTKFIXED,37.37096076368,126.72163015176,8.1608,22.3000,0.3647,0.2816,-0.0115,-0.296506050,-1.118124475,33.712011853,0.4164,0.2937,0.5589,0.1136,0.0946,0.0836,0.2655,0.2400,5.1444,0f000001,0*688a566e\n\t", "INSPVAXA,USB3,0,49.5,FINESTEERING,2107,281394.850,02000000,471d,15824;INS_ALIGNMENT_COMPLETE,INS_RTKFIXED,37.37096245961,126.72163173093,8.1552,22.3000,0.3611,0.2897,0.0065,-0.395039042,-1.114938757,33.806057490,0.4164,0.2937,0.5589,0.1136,0.0946,0.0836,0.2655,0.2400,5.1444,0f000001,0*207a4651\n\t", "INSPVAXA,USB3,0,47.5,FINESTEERING,2107,281395.850,02000000,471d,15824;INS_ALIGNMENT_COMPLETE,INS_RTKFIXED,37.37096587417,126.72163486610,8.1446,22.3000,0.3698,0.2924,-0.0143,-0.371056293,-0.946940262,33.969984358,0.4152,0.2922,0.5549,0.1139,0.0950,0.0842,0.2655,0.2400,5.1444,0f000001,0*416a3ff6\n\t", "INSPVAXA,USB3,0,47.5,FINESTEERING,2107,281396.350,02000000,471d,15824;INS_ALIGNMENT_COMPLETE,INS_RTKFIXED,37.37096753829,126.72163640742,8.1378,22.3000,0.3398,0.2681,-0.0087,-0.164596770,-1.133388969,33.930144164,0.4145,0.2919,0.5524,0.1132,0.0937,0.0831,0.2654,0.2399,5.1441,0f000001,0*c9e3845c\n\t", "INSPVAXA,USB3,0,47.5,FINESTEERING,2107,281396.850,02000000,471d,15824;INS_ALIGNMENT_COMPLETE,INS_RTKFIXED,37.37096924651,126.72163797428,8.1309,22.3000,0.3574,0.2705,-0.0020,-0.147004218,-0.814443066,33.921255816,0.4145,0.2919,0.5524,0.1132,0.0937,0.0831,0.2654,0.2399,5.1441,0f000001,0*98005433\n\t", "INSPVAXA,USB3,0,49.5,FINESTEERING,2107,281397.350,02000000,471d,15824;INS_ALIGNMENT_COMPLETE,INS_RTKFIXED,37.37097094637,126.72163952751,8.1230,22.3000,0.3568,0.2763,-0.0303,-0.204424116,-0.677389898,33.930384401,0.4166,0.2976,0.5621,0.1134,0.0950,0.0840,0.2655,0.2398,5.1447,0f000001,0*229e290a\n\t", "INSPVAXA,USB3,0,49.5,FINESTEERING,2107,281397.850,02000000,471d,15824;INS_ALIGNMENT_COMPLETE,INS_RTKFIXED,37.37097267317,126.72164110503,8.1156,22.3000,0.3644,0.2601,0.0030,-0.207601893,-0.850493393,33.903346021,0.4166,0.2976,0.5621,0.1134,0.0950,0.0840,0.2655,0.2398,5.1447,0f000001,0*99e15a33\n\t", "INSPVAXA,USB3,0,47.0,FINESTEERING,2107,281398.350,02000000,471d,15824;INS_ALIGNMENT_COMPLETE,INS_RTKFIXED,37.37097438871,126.72164266550,8.1100,22.3000,0.3561,0.2764,-0.0101,-0.236656715,-0.969278432,33.883238770,0.4175,0.2995,0.5669,0.1134,0.0951,0.0842,0.2654,0.2398,5.1455,0f000001,0*71e938c6\n\t", "INSPVAXA,USB3,0,47.0,FINESTEERING,2107,281398.850,02000000,471d,15824;INS_ALIGNMENT_COMPLETE,INS_RTKFIXED,37.37097610679,126.72164421082,8.1028,22.3000,0.3606,0.2818,-0.0239,-0.382752172,-0.849124601,34.007737280,0.4175,0.2995,0.5669,0.1134,0.0951,0.0842,0.2654,0.2398,5.1455,0f000001,0*8bea9a1b\n\t", "INSPVAXA,USB3,0,48.0,FINESTEERING,2107,281399.350,02000000,471d,15824;INS_ALIGNMENT_COMPLETE,INS_RTKFIXED,37.37097781437,126.72164579637,8.0962,22.3000,0.3464,0.2856,-0.0229,-0.220443352,-0.638082090,34.139023670,0.4187,0.3008,0.5721,0.1133,0.0950,0.0843,0.2654,0.2397,5.1467,0f000001,0*4de46431\n\t", "INSPVAXA,USB3,0,48.0,FINESTEERING,2107,281399.850,02000000,471d,15824;INS_ALIGNMENT_COMPLETE,INS_RTKFIXED,37.37097954920,126.72164741016,8.0894,22.3000,0.3776,0.2848,-0.0077,-0.220802619,-0.919793940,34.236212275,0.4187,0.3008,0.5721,0.1133,0.0950,0.0843,0.2654,0.2397,5.1467,0f000001,0*1294b3ed\n\t", "INSPVAXA,USB3,0,51.0,FINESTEERING,2107,281400.350,02000000,471d,15824;INS_ALIGNMENT_COMPLETE,INS_RTKFIXED,37.37098127121,126.72164900828,8.0835,22.3000,0.3512,0.2798,-0.0167,-0.348314510,-1.071908763,34.359634607,0.4200,0.3034,0.5796,0.1133,0.0952,0.0845,0.2654,0.2397,5.1479,0f000001,0*0d7d68ff\n\t", "INSPVAXA,USB3,0,47.5,FINESTEERING,2107,281401.350,02000000,471d,15824;INS_ALIGNMENT_COMPLETE,INS_RTKFIXED,37.37098468255,126.72165224111,8.0693,22.3000,0.3522,0.2654,-0.0166,-0.377347631,-0.696818935,34.675390534,0.4199,0.3031,0.5827,0.1133,0.0950,0.0845,0.2653,0.2397,5.1493,0f000001,0*9d8e74ce\n\t", "INSPVAXA,USB3,0,47.5,FINESTEERING,2107,281401.850,02000000,471d,15824;INS_ALIGNMENT_COMPLETE,INS_RTKFIXED,37.37098640066,126.72165387594,8.0604,22.3000,0.3637,0.3053,-0.0327,-0.270135271,-0.804168366,34.795363793,0.4199,0.3031,0.5827,0.1133,0.0950,0.0845,0.2653,0.2397,5.1493,0f000001,0*da64b754\n\t", "INSPVAXA,USB3,0,50.5,FINESTEERING,2107,281402.350,02000000,471d,15824;INS_ALIGNMENT_COMPLETE,INS_RTKFIXED,37.37098814311,126.72165553313,8.0529,22.3000,0.3514,0.2761,-0.0227,-0.415994366,-1.222362731,34.800018159,0.4207,0.3056,0.5893,0.1133,0.0953,0.0846,0.2653,0.2396,5.1507,0f000001,0*f3097738\n\t", "INSPVAXA,USB3,0,50.5,FINESTEERING,2107,281402.850,02000000,471d,15824;INS_ALIGNMENT_COMPLETE,INS_RTKFIXED,37.37098982425,126.72165714706,8.0452,22.3000,0.3664,0.2820,-0.0237,-0.514294339,-1.108715950,34.873142980,0.4207,0.3056,0.5893,0.1133,0.0953,0.0846,0.2653,0.2396,5.1507,0f000001,0*3533bd5f\n\t", "INSPVAXA,USB3,0,46.5,FINESTEERING,2107,281403.350,02000000,471d,15824;INS_ALIGNMENT_COMPLETE,INS_RTKFIXED,37.37099150836,126.72165880250,8.0350,22.3000,0.3619,0.2923,-0.0388,-0.135694474,-1.036034406,34.888546976,0.4207,0.3066,0.5937,0.1132,0.0955,0.0846,0.2653,0.2396,5.1519,0f000001,0*7db2ed89\n\t", "INSPVAXA,USB3,0,45.5,FINESTEERING,2107,281404.350,02000000,471d,15824;INS_ALIGNMENT_COMPLETE,INS_RTKFIXED,37.37099493279,126.72166212564,8.0179,22.3000,0.3493,0.2735,-0.0199,-0.409952245,-1.106661495,34.971995764,0.4183,0.3008,0.5856,0.1131,0.0947,0.0839,0.2651,0.2395,5.1529,0f000001,0*541bafca\n\t", "INSPVAXA,USB3,0,45.5,FINESTEERING,2107,281404.850,02000000,471d,15824;INS_ALIGNMENT_COMPLETE,INS_RTKFIXED,37.37099660227,126.72166374929,8.0125,22.3000,0.3621,0.2956,-0.0286,-0.267167833,-0.753528343,34.912800683,0.4183,0.3008,0.5856,0.1131,0.0947,0.0839,0.2651,0.2395,5.1529,0f000001,0*d35c1563\n\t", "INSPVAXA,USB3,0,47.0,FINESTEERING,2107,281405.350,02000000,471d,15824;INS_ALIGNMENT_COMPLETE,INS_RTKFIXED,37.37099831104,126.72166542304,8.0059,22.3000,0.3575,0.2905,-0.0163,-0.253871476,-0.573976572,34.788811837,0.4180,0.3006,0.5851,0.1139,0.0957,0.0850,0.2651,0.2394,5.1534,0f000001,0*ea0daca7\n\t", "INSPVAXA,USB3,0,47.0,FINESTEERING,2107,281405.850,02000000,471d,15824;INS_ALIGNMENT_COMPLETE,INS_RTKFIXED,37.37100000968,126.72166711041,8.0001,22.3000,0.3748,0.2860,-0.0242,-0.088360721,-0.852531468,34.685538696,0.4180,0.3006,0.5851,0.1139,0.0957,0.0850,0.2651,0.2394,5.1534,0f000001,0*79314379\n\t", "INSPVAXA,USB3,0,49.0,FINESTEERING,2107,281406.350,02000000,471d,15824;INS_ALIGNMENT_COMPLETE,INS_RTKFIXED,37.37100175880,126.72166880875,7.9944,22.3000,0.3745,0.2914,-0.0180,-0.078489468,-1.009185003,34.665355987,0.4165,0.2969,0.5768,0.1147,0.0961,0.0860,0.2650,0.2394,5.1543,0f000001,0*41bb7608\n\t", "INSPVAXA,USB3,0,49.0,FINESTEERING,2107,281407.350,02000000,471d,15824;INS_ALIGNMENT_COMPLETE,INS_RTKFIXED,37.37100512322,126.72167206883,7.9829,22.3000,0.3677,0.2809,-0.0383,0.055269502,-0.871990606,34.333614581,0.4159,0.2956,0.5723,0.1160,0.0974,0.0881,0.2649,0.2393,5.1550,0f000001,0*e297d913\n\t", "INSPVAXA,USB3,0,49.0,FINESTEERING,2107,281407.850,02000000,471d,15824;INS_ALIGNMENT_COMPLETE,INS_RTKFIXED,37.37100682475,126.72167368991,7.9758,22.3000,0.3450,0.2906,-0.0278,0.076806319,-0.668802116,34.237004586,0.4159,0.2956,0.5723,0.1160,0.0974,0.0881,0.2649,0.2393,5.1550,0f000001,0*eb42bcbe\n\t", "INSPVAXA,USB3,0,49.0,FINESTEERING,2107,281408.350,02000000,471d,15824;INS_ALIGNMENT_COMPLETE,INS_RTKFIXED,37.37100857076,126.72167534247,7.9736,22.3000,0.3634,0.2846,-0.0190,-0.182813493,-0.879750967,34.094650062,0.4161,0.2965,0.5711,0.1145,0.0958,0.0868,0.2649,0.2393,5.1559,0f000001,0*ba1fbbd1\n\t", "INSPVAXA,USB3,0,49.0,FINESTEERING,2107,281408.850,02000000,471d,15824;INS_ALIGNMENT_COMPLETE,INS_RTKFIXED,37.37101026525,126.72167697337,7.9727,22.3000,0.3524,0.2783,-0.0246,-0.098737305,-0.690752334,33.910631500,0.4161,0.2965,0.5711,0.1145,0.0958,0.0868,0.2649,0.2393,5.1559,0f000001,0*d5b16fe8\n\t", "INSPVAXA,USB3,0,47.5,FINESTEERING,2107,281409.350,02000000,471d,15824;INS_ALIGNMENT_COMPLETE,INS_RTKFIXED,37.37101200437,126.72167857017,7.9719,22.3000,0.3673,0.3066,-0.0244,-0.420788016,-0.858221661,33.836234761,0.4162,0.2973,0.5715,0.1138,0.0952,0.0865,0.2649,0.2392,5.1570,0f000001,0*5513fa8f\n\t", "INSPVAXA,USB3,0,49.0,FINESTEERING,2107,281410.850,02000000,471d,15824;INS_ALIGNMENT_COMPLETE,INS_RTKFIXED,37.37101714160,126.72168333239,7.9694,22.3000,0.3574,0.2819,-0.0127,-0.504237932,-0.910801054,33.584207367,0.4157,0.2969,0.5709,0.1135,0.0948,0.0862,0.2649,0.2392,5.1584,0f000001,0*1e770ccd\n\t", "INSPVAXA,USB3,0,49.0,FINESTEERING,2107,281411.350,02000000,471d,15824;INS_ALIGNMENT_COMPLETE,INS_RTKFIXED,37.37101885346,126.72168493250,7.9707,22.3000,0.3563,0.2832,-0.0055,-0.267715843,-0.919384787,33.461951362,0.4158,0.2973,0.5713,0.1134,0.0948,0.0862,0.2649,0.2392,5.1601,0f000001,0*2f0cc835\n\t", "INSPVAXA,USB3,0,49.0,FINESTEERING,2107,281411.850,02000000,471d,15824;INS_ALIGNMENT_COMPLETE,INS_RTKFIXED,
